vi "cursors list.vi"(8 "error in":errorcluster, 11 "Table":string[][](table)) -> (0 "error out":errorcluster, 3 "Cursors List":T1(array[cluster]))   [LabVIEW 2023]
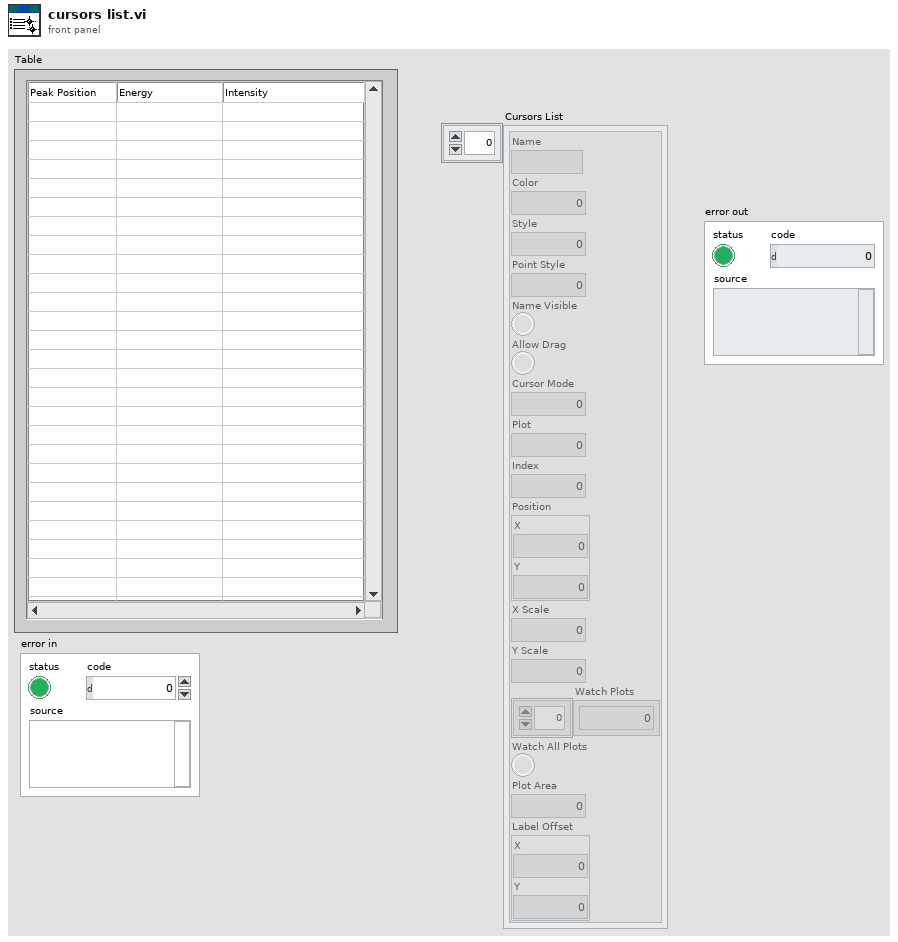
[diagram p1: front panel]
types:
  T1 = cluster{"Name":string, "Color":u32, "Style":i32, "Point Style":i32, "Name Visible":bool, "Allow Drag":bool, "Cursor Mode":u32, "Plot":i32, "Index":i32, "Position":cluster{"X":dbl, "Y":dbl}, "X Scale":u32, "Y Scale":u32, "Watch Plots":i32[], "Watch All Plots":bool, "Plot Area":i32, "Label Offset":cluster{"X":dbl, "Y":dbl}}[]
  T2 = cluster{"Name":string, "Color":u32, "Style":i32, "Point Style":i32, "Name Visible":bool, "Allow Drag":bool, "Cursor Mode":u32, "Plot":i32, "Index":i32, "Position":cluster{"X":dbl, "Y":dbl}, "X Scale":u32, "Y Scale":u32, "Watch Plots":i32[], "Watch All Plots":bool, "Plot Area":i32, "Label Offset":cluster{"X":dbl, "Y":dbl}}
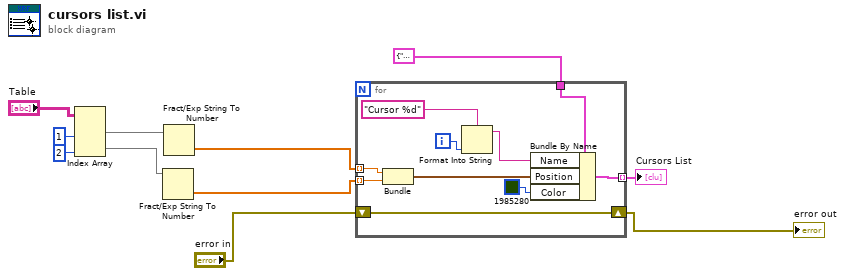
[diagram p0: block diagram]
diagram:
  n1 = Index Array(array="Table", index (col) #1=1 ("disabled index (col)"), index (col) #2=2 ("index (col)")) -> (element #1=w7:string[], element #2=w6:string[])  [unwired: 2 in]
  n2 = Fract/Exp String To Number(string=w6) -> (number=w4:dbl[])  [unwired: 3 in, 1 out]
  n3 = Fract/Exp String To Number(string=w7) -> (number=w5:dbl[])  [unwired: 3 in, 1 out]
  n4 = for {
    tunnel: w5 -> [w19] mode=indexing
    tunnel: w4 -> [w18] mode=indexing
    tunnel: T2 {"Name"="", "Color"=16776704, "Style"=4, "Point Style"=13, "Name Visible"=FALSE, "Allow Drag"=TRUE, "Cursor Mode"=0, "Plot"=0, "Index"=0, "Position"={"X"=0.0, "Y"=0.0}, "X Scale"=0, "Y Scale"=0, "Watch Plots"=[], "Watch All Plots"=FALSE, "Plot Area"=0, "Label Offset"={"X"=0.0, "Y"=0.0}} -> [w17]
    tunnel: [w13] -> w1 mode=indexing
    shift-right: [w12] -> w2
    shift-left: "error in" -> [w12]
    i -> [w20]
    n5 = Bundle(w19, w18) -> (w14:cluster{dbl, dbl})  [unwired: 1 in]
    n6 = Format Into String(format string="Cursor %d", w20) -> (resulting string=w16:string)  [unwired: 2 in, 1 out]
    n7 = Bundle By Name(cluster=w17, "Name"=w16, "Position"=w14, "Color"=u32 1985280) -> (w13:T2)
  }
  "error out" <- w2
  "Cursors List" <- w1
